vi "_attribute_write.vi"(1 "Boolean in":bool, 4 "String in":string, 5 "Int64 in":i64, 6 "Repeated Capability":string, 7 "Int32 in":i32, 8 "error in":errorcluster caption="error in (no error)", 9 "Double in":dbl, 10 "Attribute ID":string, 11 "VISA resource name":refnum<visa-resource-name>) -> (0 "error out":errorcluster, 3 "VISA resource name out":refnum<visa-resource-name>)   [LabVIEW 2022 SP3, in "hmp4000_rsidr_core.lvlib"]
uses:
  hmp4000_rsidr_core.lvlib
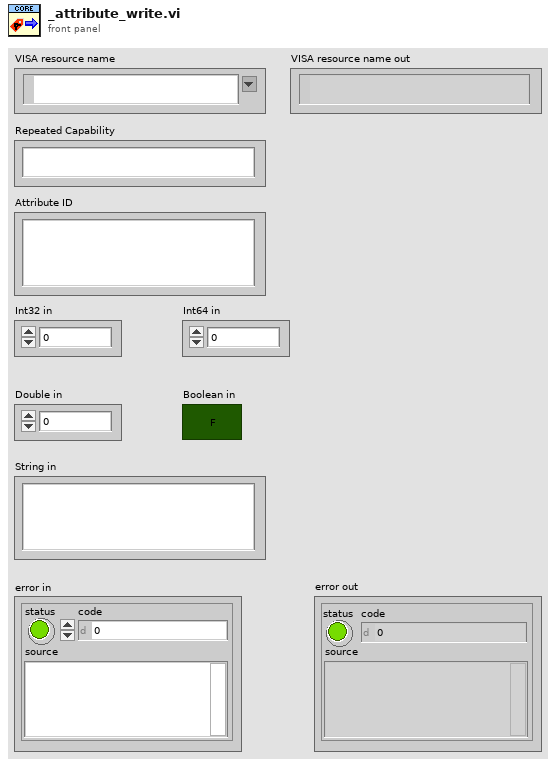
[diagram p1: front panel]
types:
  T1 = typedef "hmp4000_rsidr_core.lvlib/type_Attribute.ctl" = cluster{"Identifier":string, "Descriptive Name":string, "Data Type":T2, "Command":string, "Access":T3, "Range Table":string, "Read Callback":string, "Write Callback":string, "Supported Models":string, "Instrument Options":string, "Index":i32, "OPC Wait":bool, "No Status Check":bool, "Cache Only":bool}
  T2 = typedef "hmp4000_rsidr_core.lvlib/type_Attribute_Data_Type.ctl" = enum16{"Integer 32", "Double", "String", "Boolean", "None", "Integer 64", "RawString"}
  T3 = typedef "hmp4000_rsidr_core.lvlib/type_ReadWriteAccess.ctl" = enum16{"Read Only", "Write Only", "Read/Write"}
  T4 = typedef "hmp4000_rsidr_core.lvlib/type_Session_Data.ctl" = cluster{"IDN string":string, "Instrument FW":string, "Instr type":string, "Instr type for err. msg.":string, "Installed Options":string[], "Ignore Error Messages":string, "Logging params":variant, "OPC Timeout":i32, "VISA Timeout":i32, "STB Poll VISA Timeout":i32, "Additional Flags":i32, "Wait Before Read":i32, "Wait Before Write":i32, "Option String Flags":i32, "IO Segment Size":i64, "VISA Access Mode":T5, "Interface Type":T6, "OPC Wait Mode":T7, "Bin Float Number  Format":T8, "Bin Integer Number Format":T9, "Simulate":bool, "VXIcapable":bool, "Duplicate Session":bool, "Add LF to Write":bool, "Logging":bool, "Fast Sweep":bool, "Query Instrument Status":bool, "Check Range":bool, "Check Options":bool}
  T5 = typedef "hmp4000_rsidr_core.lvlib/type_VisaAccessMode.ctl" = u16
  T6 = typedef "hmp4000_rsidr_core.lvlib/type_InterfaceType.ctl" = enum16{"Unknown", "GPIB", "VXI", "GPIB_VXI", "ASRL", "PXI", "TCPIP", "USB", "SOCKET"}
  T7 = typedef "hmp4000_rsidr_core.lvlib/type_OPC_Wait_Mode.ctl" = enum16{"STBpolling", "STBpollingSlow", "STBpollingSuperSlow", "ServiceRequest", "OPCquery"}
  T8 = typedef "hmp4000_rsidr_core.lvlib/type_Binary_Float_Number_Format.ctl" = enum16{"Float_4_Bytes_Swapped", "Float_4_Bytes", "Double_8_Bytes_Swapped", "Double_8_Bytes"}
  T9 = typedef "hmp4000_rsidr_core.lvlib/type_Binary_Integer_Number_Format.ctl" = enum16{"Int32_4_Bytes_Swapped", "Int32_4 Bytes", "Int16_2_Bytes_Swapped", "Int16_2_Bytes"}
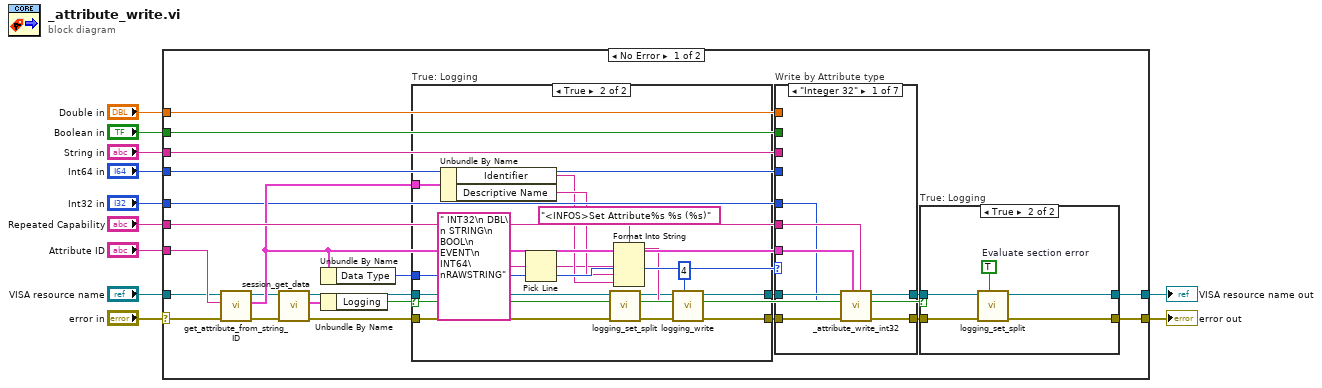
[diagram p0: block diagram]
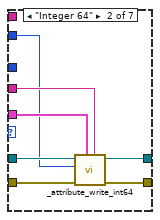
[diagram p4: hidden frame]
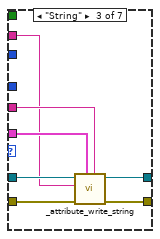
[diagram p5: hidden frame]
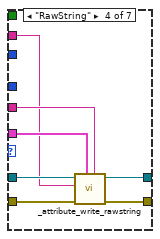
[diagram p6: hidden frame]
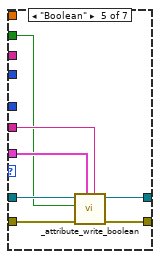
[diagram p7: hidden frame]
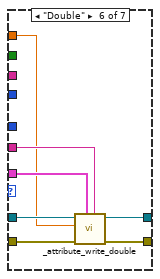
[diagram p8: hidden frame]
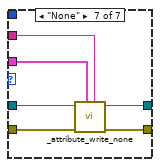
[diagram p9: hidden frame]
diagram:
  n1 = case shown="No Error" "error in" {
    selector: "error in" -> [w22 w107]
    tunnel: "VISA resource name" -> [w13 w108]
    tunnel: "Repeated Capability" -> [w34 _]
    tunnel: [w29 w108] -> w9
    tunnel: [w30 w107] -> w8
    tunnel: "Attribute ID" -> [w20 _]
    tunnel: "Int32 in" -> [w18 _]
    tunnel: "Int64 in" -> [w17 _]
    tunnel: "String in" -> [w16 _]
    tunnel: "Boolean in" -> [w15 _]
    tunnel: "Double in" -> [w14 _]
    frame No Error {
      n2 = call "get_attribute_from_string_ID.vi"("error in"=w22, "Attribute ID in"=w20, "VISA resource name"=w13) -> ("error out"=w21:errorcluster, "Attribute out"=w19:T1, "VISA resource name out"=w12:refnum<visa-resource-name>)  [unwired: 6 in]
      n3 = call "session_get_data.vi"("error in"=w21, "VISA resource name"=w12) -> ("error out"=w27:errorcluster, "Session User Data out"=w23:T4, "VISA resource name out"=w26:refnum<visa-resource-name>)  [unwired: 6 in, 1 out]
      n4 = Unbundle By Name(w19) -> ("Data Type"=w33:T2)
      n5 = Unbundle By Name(w23) -> ("Logging"=w28:bool)
      n6 = case "True: Logging" shown="True" w28 {
        tunnel: w27 -> [w43 w49]
        tunnel: [w43 w45] -> w25
        tunnel: w19 -> [_ w58]
        tunnel: w26 -> [w42 w48]
        tunnel: [w42 w44] -> w24
        tunnel: w33 -> [_ w52]
        frame False {
        }
        frame True {
          n7 = Unbundle By Name(w58) -> ("Identifier"=w55:string, "Descriptive Name"=w56:string)
          n8 = Pick Line(multi-line string=" INT32\n DBL\n STRING\n BOOL\n EVENT\n INT64\nRAWSTRING", line index=w52) -> (output string=w51:string)  [unwired: 1 in]
          n9 = call "logging_set_split.vi"("error in"=w49, "VISA resource name"=w48) -> ("error out"=w47:errorcluster, "VISA resource name out"=w46:refnum<visa-resource-name>)  [unwired: 8 in]
          n10 = Format Into String(format string="<INFOS>Set Attribute%s %s (%s)", w51, w56, w55) -> (resulting string=w54:string)  [unwired: 2 in, 1 out]
          n11 = call "logging_write.vi"("Add call chain offset\n(No call chain)"=4 ("Add call chain offset\n(No call chain)"), "error in"=w47, "String to write"=w54, "VISA resource name"=w46) -> ("error out"=w45:errorcluster, "VISA resource name out"=w44:refnum<visa-resource-name>)  [unwired: 6 in]
        }
      }
      n12 = case "Write by Attribute type" shown="\"Integer 32\"" w33 {
        tunnel: w19 -> [w61 w67 w74 w81 w88 w99 w102]
        tunnel: w24 -> [w65 w72 w79 w86 w93 w98 w106]
        tunnel: w25 -> [w64 w71 w78 w85 w92 w95 w101]
        tunnel: w34 -> [w60 w68 w75 w82 w89 w100 w103]
        tunnel: [w63 w70 w77 w84 w91 w96 w105] -> w31
        tunnel: [w62 w69 w76 w83 w90 w97 w104] -> w32
        tunnel: w18 -> [w59 _ _ _ _ _ _]
        tunnel: w17 -> [_ w66 _ _ _ _ _]
        tunnel: w16 -> [_ _ w73 w80 _ _ _]
        tunnel: w15 -> [_ _ _ _ w87 _ _]
        tunnel: w14 -> [_ _ _ _ _ w94 _]
        frame "Integer 32" {
          n13 = call "_attribute_write_int32.vi"("Repeated Capability"=w60, "Attribute"=w61, "error in"=w64, "Int32 in"=w59, "VISA resource name"=w65) -> ("error out"=w62:errorcluster, "VISA resource name out"=w63:refnum<visa-resource-name>)  [unwired: 5 in]
        }
        frame "Integer 64" {
          n14 = call "_attribute_write_int64.vi"("Repeated Capability"=w68, "Attribute"=w67, "error in"=w71, "Int64 in"=w66, "VISA resource name"=w72) -> ("error out"=w69:errorcluster, "VISA resource name out"=w70:refnum<visa-resource-name>)  [unwired: 5 in]
        }
        frame "String" {
          n15 = call "_attribute_write_string.vi"("Repeated Capability"=w75, "Attribute"=w74, "error in"=w78, "String in"=w73, "VISA resource name"=w79) -> ("error out"=w76:errorcluster, "VISA resource name out"=w77:refnum<visa-resource-name>)  [unwired: 5 in]
        }
        frame "RawString" {
          n16 = call "_attribute_write_rawstring.vi"("Repeated Capability"=w82, "Attribute"=w81, "error in"=w85, "Raw String in"=w80, "VISA resource name"=w86) -> ("error out"=w83:errorcluster, "VISA resource name out"=w84:refnum<visa-resource-name>)  [unwired: 5 in]
        }
        frame "Boolean" {
          n17 = call "_attribute_write_boolean.vi"("Repeated Capability"=w89, "Attribute"=w88, "error in"=w92, "Boolean in"=w87, "VISA resource name"=w93) -> ("error out"=w90:errorcluster, "VISA resource name out"=w91:refnum<visa-resource-name>)  [unwired: 5 in]
        }
        frame "Double" {
          n18 = call "_attribute_write_double.vi"("Repeated Capability"=w100, "Attribute"=w99, "error in"=w95, "Double in"=w94, "VISA resource name"=w98) -> ("error out"=w97:errorcluster, "VISA resource name out"=w96:refnum<visa-resource-name>)  [unwired: 5 in]
        }
        frame "None" {
          n19 = call "_attribute_write_none.vi"("Repeated Capability"=w103, "Attribute"=w102, "error in"=w101, "VISA resource name"=w106) -> ("error out"=w104:errorcluster, "VISA resource name out"=w105:refnum<visa-resource-name>)  [unwired: 6 in]
        }
      }
      n20 = case "True: Logging" shown="True" w28 {
        tunnel: w32 -> [w36 w41]
        tunnel: [w36 w39] -> w30
        tunnel: w31 -> [w35 w40]
        tunnel: [w35 w38] -> w29
        frame False {
        }
        frame True {
          w37 = TRUE  # Evaluate section error
          n21 = call "logging_set_split.vi"("Evaluate section error (F)"=w37, "error in"=w41, "VISA resource name"=w40) -> ("error out"=w39:errorcluster, "VISA resource name out"=w38:refnum<visa-resource-name>)  [unwired: 7 in]
        }
      }
    }
    frame Error {
    }
  }
  "error out" <- w8
  "VISA resource name out" <- w9
